vi "Start Timer.vi"(8 "error in (no error)":errorcluster, 9 "Timeout (1000)":i32=1000, 10 "Timer (Absolute)":i32(ring) items=["Absolute", "Relative"], 11 "VISA resource name":refnum<visa-resource-name>) -> (0 "error out":errorcluster, 3 "VISA resource name out":refnum<visa-resource-name>)   [LabVIEW 2020, in "Rohde&Schwarz CMXP Base.lvlib"]
doc: "This VI starts a timer.\n\nAttributes:\nRSCMXPBASE_ATTR_SET_ABSOLUTE_TIMER\nRSCMXPBASE_ATTR_SET_RELATIVE_TIMER\n\nRemote-control commands:\nSYSTem:TIME:HRTimer:ABSolute\nSYSTem:TIME:HRTimer:RELative"
uses:
  <instrlib>/Rohde&Schwarz CMXP Base/Rohde&Schwarz CMXP Base.lvlib
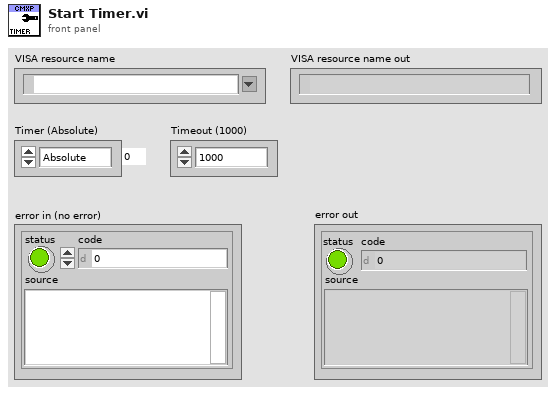
[diagram p1: front panel]
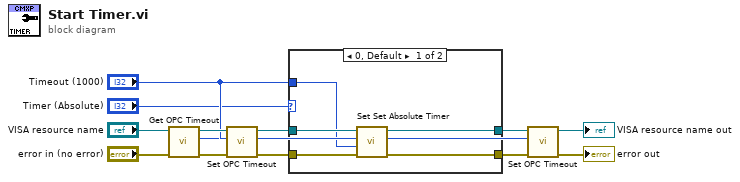
[diagram p0: block diagram]
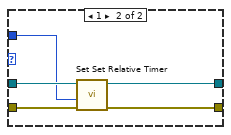
[diagram p2: hidden frame]
diagram:
  n1 = call <instrlib>:"Get OPC Timeout.vi"("error in (no error)"="error in (no error)", "VISA resource name"="VISA resource name") -> ("error out"=w11:errorcluster, "OPC Timeout"=w1:i32, "VISA resource name out"=w10:refnum<visa-resource-name>)  [unwired: 7 in]
  n2 = call <instrlib>:"Set OPC Timeout.vi"("error in (no error)"=w11, "OPC Timeout"="Timeout (1000)", "VISA resource name"=w10) -> ("error out"=w9:errorcluster, "VISA resource name out"=w8:refnum<visa-resource-name>)  [unwired: 7 in]
  n3 = case shown="0, Default" "Timer (Absolute)" {
    tunnel: w9 -> [w18 w23]
    tunnel: w8 -> [w17 w22]
    tunnel: [w16 w21] -> w7
    tunnel: [w15 w20] -> w6
    tunnel: "Timeout (1000)" -> [w14 w19]
    frame 0, Default {
      n4 = call "Set Set Absolute Timer"("error in (no error)"=w18, "Set Absolute Timer (0)"=w14, "instrument handle"=w17) -> ("error out"=w16:errorcluster, "instrument handle out"=w15:refnum<visa-resource-name>)  [unwired: 7 in]
    }
    frame 1 {
      n5 = call "Set Set Relative Timer"("error in (no error)"=w23, "Set Relative Timer (0)"=w19, "instrument handle"=w22) -> ("error out"=w21:errorcluster, "instrument handle out"=w20:refnum<visa-resource-name>)  [unwired: 7 in]
    }
  }
  n6 = call <instrlib>:"Set OPC Timeout.vi"("error in (no error)"=w7, "OPC Timeout"=w1, "VISA resource name"=w6) -> ("error out"=→"error out":errorcluster, "VISA resource name out"=→"VISA resource name out":refnum<visa-resource-name>)  [unwired: 7 in]
